vi "sorting array.vi"() -> ()   [LabVIEW 2020]
uses:
  65aa39dc-c2ef-4a1f-86c4-5c1ef9422506.vi
  87a8b836-6717-48af-9df3-1bedfa631d5c.vi
  773a2108-dbf7-4d00-9ada-8d0c01f718e6.vi
  995066d3-160f-4ac6-a8b7-62b98a26110a.vi
  <vilib>/Comparison/Less/Less Functor/Less Functor.lvclass
panel:
  out "all ok?":bool
  out "dup removed":i32
  out "dobble sizesize(s)":i32
  out "finished size(s)":i32
  out "finished":i32[](array[numeric])
  out "dup removed":i32[](array[numeric])
  out "sorted array":i32[](array[numeric])
  out "shuffled array":i32[](array[numeric])
  out "org":i32[](array[numeric])
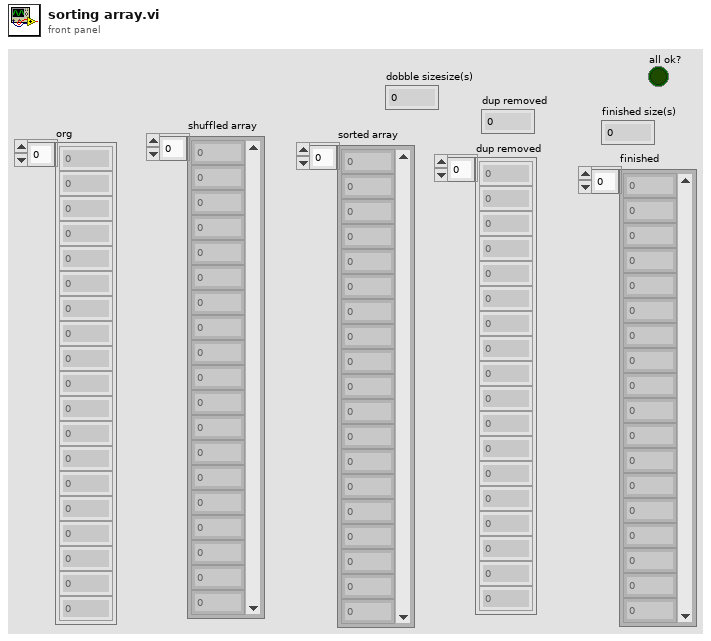
[diagram p1: front panel]
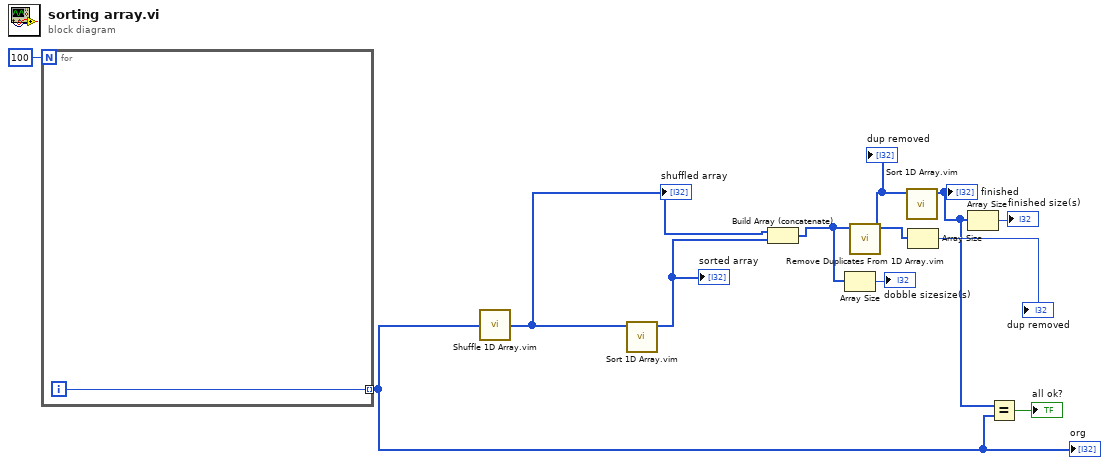
[diagram p0: block diagram]
diagram:
  n1 = for {
    N: 100 -> [_]
    tunnel: [w12] -> w2 mode=indexing
    i -> [w12]
  }
  "org" <- w2
  n2 = call "Shuffle 1D Array.vim"("array"=w2) -> ("shuffled array"=w9:i32[])  [unwired: 4 in]
  "shuffled array" <- w9
  n3 = call "Sort 1D Array.vim"("unsorted array"=w9) -> ("sorted array"=w10:i32[])  [unwired: 10 in]
  "sorted array" <- w10
  n4 = Build Array (concatenate)(w9, w10) -> (w7:i32[])
  n5 = Array Size(array=w7) -> (size(s)=→"dobble sizesize(s)":i32)
  n6 = call "Remove Duplicates From 1D Array.vim"("array"=w7) -> ("array with duplicates removed"=w5:i32[])  [unwired: 10 in]
  "dup removed" <- w5
  n7 = call "Sort 1D Array.vim"("unsorted array"=w5) -> ("sorted array"=w3:i32[])  [unwired: 10 in]
  "finished" <- w3
  n8 = Array Size(array=w5) -> (size(s)=→"dup removed":i32)
  n9 = Array Size(array=w3) -> (size(s)=→"finished size(s)":i32)
  n10 = Equal?(x=w3, y=w2) -> (x = y?=→"all ok?":bool)
